vi "NI VeriStand - Open Command Line Notification (Macro Player).vi"(8 "error in (no error)":errorcluster, 11 "MacroPlayer in":T2) -> (0 "error out":errorcluster, 2 "CommandLine Refs":T1, 3 "MacroPlayer out":T2)   [LabVIEW 2020, in "NI_VS MacroPlayerAPI.lvlib"]
doc: "Opens a reference to the command line of the Macro Player tool. Opening this reference enables you to use the Get Macro Player Command Lines VI to read the commands the VeriStand Gateway sends to the RT target or desktop PC. This VI also returns a user event that you can register and wire to an Event structure."
uses:
  <vilib>/NI VeriStand/Execution/MacroPlayer/NI_VS MacroPlayerAPI.lvlib
  <vilib>/NI VeriStand/Execution/MacroPlayer/MacroPlayerAPI.ctl
  NationalInstruments.VeriStand.ClientAPI
  <vilib>/NI VeriStand/Execution/MacroPlayer/CommandLine Refs.ctl
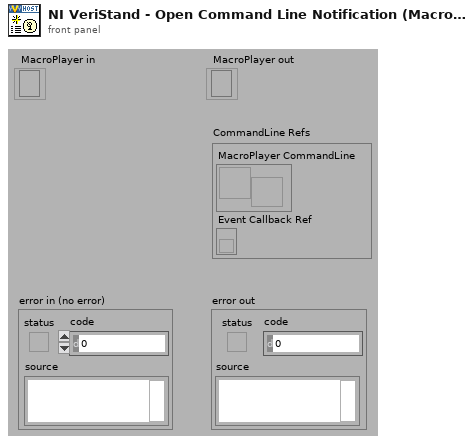
[diagram p1: front panel]
types:
  T1 = typedef "NI_VS MacroPlayerAPI.lvlib/CommandLine Refs.ctl" = cluster{"MacroPlayer CommandLine":refnum<user-event>, "Event Callback Ref":refnum<k27>}
  T2 = typedef "NI_VS MacroPlayerAPI.lvlib/MacroPlayerAPI.ctl" = refnum<k24>
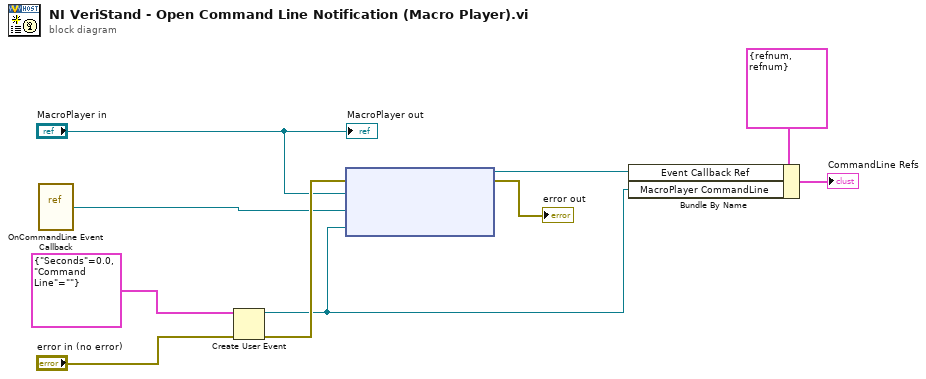
[diagram p0: block diagram]
diagram:
  n1 = vi-ref <vilib>:"OnCommandLine Event Callback.vi"() -> ("vi reference"=w1:refnum<vi>)
  n2 = Create User Event(user event datatype=cluster{"Seconds":dbl, "Command Line":string} {"Seconds"=0.0, "Command Line"=""} ("output cluster"), error in="error in (no error)") -> (user event=w4:refnum<user-event>, error out=w10:errorcluster)
  n3 = node(w10, "MacroPlayer in", w1, w4) -> (w5:refnum<k27>, →"error out":errorcluster)  [unwired: 1 in]
  n4 = Bundle By Name(cluster=T1 {"MacroPlayer CommandLine"=refnum, "Event Callback Ref"=refnum} ("CommandLine Refs"), "Event Callback Ref"=w5, "MacroPlayer CommandLine"=w4) -> (→"CommandLine Refs":T1)
  "MacroPlayer out" <- "MacroPlayer in"
